vi "OpenFpga.vi"(8 "error in (no error)":errorcluster, 11 "FpgaInterface in":refnum<class "FpgaInterface.lvclass">) -> (0 "error out":errorcluster, 3 "FpgaInterface out":refnum<class "FpgaInterface.lvclass">)   [LabVIEW 2017, in "FpgaInterface.lvclass"]
uses:
  FpgaInterface.lvclass
  <vilib>/rvi/interface/nirviReadWriteControl/nirviReadWriteControl.xnode
  NiFpgaLv.dll
  <vilib>/Utility/error.llb/Error Cluster From Error Code.vi
  <vilib>/rvi/interface/Simulation/niFpgaSimulationCallBeginRW.vi
  <vilib>/rvi/errors/niLvFpgaAdjustHostInterfaceError.vi
  <vilib>/userdefined/Silver/nirio_resource_slv.ctl
panel:
  in  "resource name":T1="RIO0"
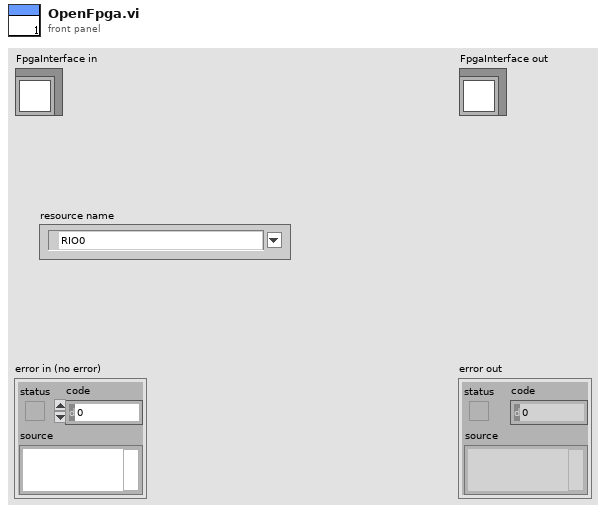
[diagram p1: front panel]
types:
  T1 = typedef "nirio_resource_slv.ctl" = tag
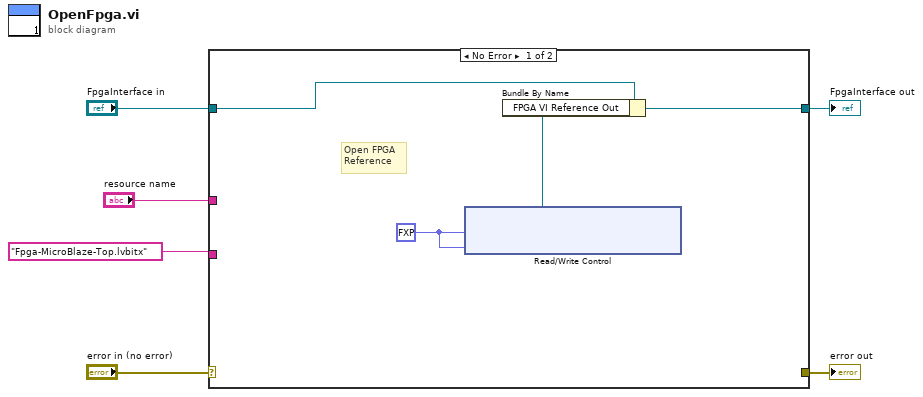
[diagram p0: block diagram]
diagram:
  n1 = case shown="No Error" "error in (no error)" {
    selector: "error in (no error)" -> [w12 w16]
    tunnel: [w11 w16] -> w5
    tunnel: [w10 w15] -> w3
    tunnel: "FpgaInterface in" -> [w9 w15]
    tunnel: "resource name" -> [w14 _]
    tunnel: "Fpga-MicroBlaze-Top.lvbitx" ("Bitfile Name") -> [w13 _]
    frame No Error {
      w7 = fxp<+,4,4> 15.0 ("d_microblaze_i\\AXI_STR_RXD_tkeep")
      # "Open FPGA\nReference"
      n2 = Bundle By Name(cluster=w9) -> (w10:refnum<class "FpgaInterface.lvclass">, "FPGA VI Reference Out"=w8:refnum<k20>)
      n3 = xnode "Read/Write Control"("FPGA VI Reference In"=w8, "d_microblaze_i\\AXI_STR_RXD_tkeep"=w7, "d_microblaze_i\\AXI_STR_RXD_1_tkeep"=w7) -> ()  [unwired: 1 in, 2 out]
    }
    frame Error {
    }
  }
  "error out" <- w5
  "FpgaInterface out" <- w3
